vi "Output Resistance.vi"(6 "Output Enabled":bool=TRUE, 7 "Impedance Compensation (0: None)":i32(ring) items=["None", "2-wire", "4-wire"], 8 "error in":errorcluster, 9 "Output Type (0: DC Volts)":i32(ring)=8 items=["DC Volts", "AC Volts", "DC Current", "AC Current", "DC Power", "AC Power", "Dual DC Volts", "Dual AC Volts", "Resistance"], 10 "Resistance (1900.0 Ohm)":dbl=1900.0, 11 "COM Port":string="COM3") -> (0 "error out":errorcluster, 3 "VISA resource name out":refnum<visa-resource-name>)   [LabVIEW 2013]
uses:
  <instrlib>/Fluke 5080/Fluke 5080.lvlib
panel:
  in  "Delay Time (s)":dbl=0.5
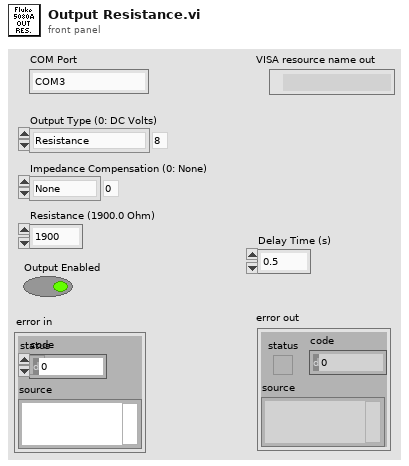
[diagram p1: front panel]
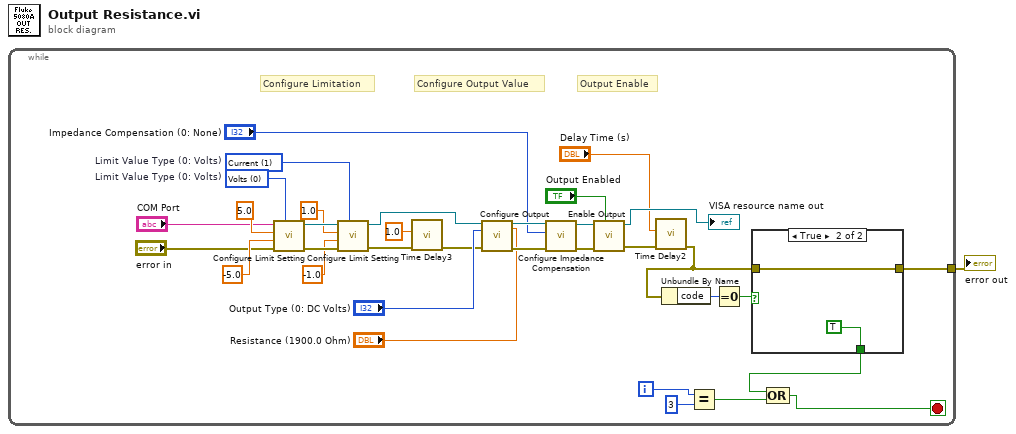
[diagram p0: block diagram]
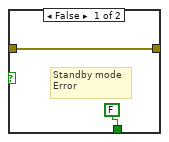
[diagram p2: hidden frame]
diagram:
  n1 = while {
    tunnel: [w2] -> w1
    i -> [w7]
    stop <- w4 stop-if-true
    w24 = 1 items=["Volts", "Current"]  # Limit Value Type (0: Volts)
    w25 = 0 items=["Volts", "Current"]  # Limit Value Type (0: Volts)
    # "Output Enable"
    # "Configure Output Value"
    # "Configure Limitation"
    n2 = call <instrlib>:"Configure Limit Setting.vi"("Limit Value Type (0: Volts)"=w25, "error in (no error)"="error in", "- Limit Value (-5)"=-5.0, "+ Limit Value (5)"=5.0, "VISA resource name"="COM Port") -> ("error out"=w26:errorcluster, "VISA resource name out"=w27:refnum<visa-resource-name>)  [unwired: 5 out]
    n3 = call <instrlib>:"Configure Limit Setting.vi"("Limit Value Type (0: Volts)"=w24, "error in (no error)"=w26, "- Limit Value (-5)"=-1.0, "+ Limit Value (5)"=1.0, "VISA resource name"=w27) -> ("error out"=w14:errorcluster, "VISA resource name out"=w12:refnum<visa-resource-name>)  [unwired: 5 out]
    n4 = call "Time Delay3"("error in (no error)"=w14, "Delay Time (s)"=1.0) -> ("error out"=w13:errorcluster)  [unwired: 9 in]
    n5 = call <instrlib>:"Configure Output.vi"("VISA resource name"=w12, "Resistance (1900.0 Ohm)"="Resistance (1900.0 Ohm)", "Output Type (0: DC Volts)"="Output Type (0: DC Volts)", "error in (no error)"=w13) -> ("VISA resource name out"=w34:refnum<visa-resource-name>, "error out"=w33:errorcluster)  [unwired: 6 in, 4 out]
    n6 = call <instrlib>:"Configure Impedance Compensation.vi"("error in (no error)"=w33, "Impedance Compensation (0: None)"="Impedance Compensation (0: None)", "VISA resource name"=w34) -> ("error out"=w29:errorcluster, "VISA resource name out"=w30:refnum<visa-resource-name>)  [unwired: 7 out]
    n7 = call <instrlib>:"Enable Output.vi"("Output Enabled (T: Enable)"="Output Enabled", "error in (no error)"=w29, "VISA resource name"=w30) -> ("error out"=w16:errorcluster, "VISA resource name out"=→"VISA resource name out":refnum<visa-resource-name>)  [unwired: 7 out]
    n8 = call "Time Delay2"("error in (no error)"=w16, "Delay Time (s)"="Delay Time (s)") -> ("error out"=w3:errorcluster)  [unwired: 9 in]
    n9 = Unbundle By Name(w3) -> ("code"=w9:i32)
    n10 = Equal?(x=w7, y=3) -> (x = y?=w8:bool)
    n11 = Equal To 0?(x=w9) -> (x = 0?=w10:bool)
    n12 = case shown="True" w10 {
      tunnel: [FALSE TRUE] -> w5
      tunnel: w3 -> [w36 w38]
      tunnel: [w36 w38] -> w2
      frame False {
        # "Standby mode\nError"
      }
      frame True {
      }
    }
    n13 = Compound Arithmetic op=OR(w5, w8) -> (w4:bool)
  }
  "error out" <- w1
